vi "Station1_Data_Log.vi"(8 "error in (no error)":errorcluster, 10 "Parameters cluster":T3, 11 "Cluster":T2) -> (0 "error out":errorcluster)   [LabVIEW 2017]
uses:
  <vilib>/addons/database/Connection.llb/Conn ObjectReference.ctl
  <vilib>/addons/database/NI_Database_API.lvlib
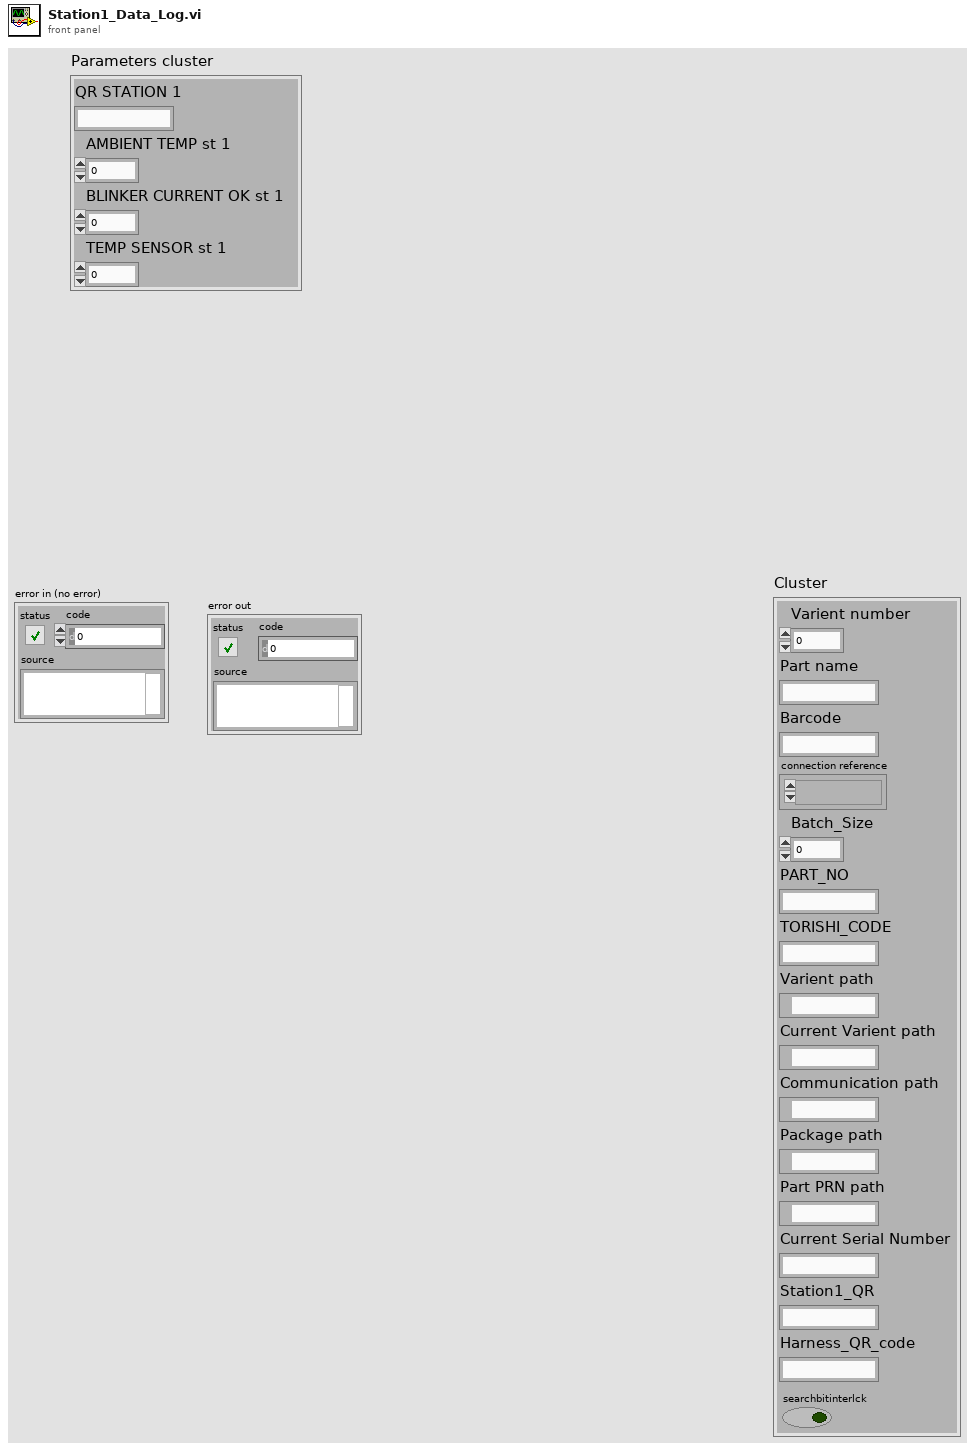
[diagram p1: front panel]
types:
  T1 = typedef "NI_Database_API.lvlib/Conn ObjectReference.ctl" = refnum<k1>
  T2 = cluster{"Varient number":u16, "Part name":string, "Barcode":string, "connection reference":T1, "Batch_Size":u16, "PART_NO":string, "TORISHI_CODE":string, "Varient path":path, "Current Varient path":path, "Communication path":path, "Package path":path, "Part PRN path":path, "Current Serial Number":string, "Station1_QR":string, "Harness_QR_code":string, "searchbitinterlck":bool}
  T3 = cluster{"QR STATION 1":string, "AMBIENT TEMP st 1":u32, "BLINKER CURRENT OK st 1":u32, "TEMP SENSOR st 1":u32}
  T4 = typedef "LVDateTimeRec.ctl" = cluster{"fractional second":dbl, "second":i32, "minute":i32, "hour":i32, "day of month":i32, "month":i32, "year":i32, "day of week":i32, "day of year":i32, "DST":i32}
  T5 = cluster{"time stamp":timestamp, string, string, "QR STATION 1":string, "Part name":string, "PART_NO":string, "TORISHI_CODE":string, string, string, "Current Serial Number":string, "Station1_QR":string, string, string, "Numeric 2":string, string, "Numeric 2":string, "Numeric 2":string, string, string, "Numeric 2":string, "Numeric 2":string, string, string, string, string, string, string, string, string, string, string, string, string}
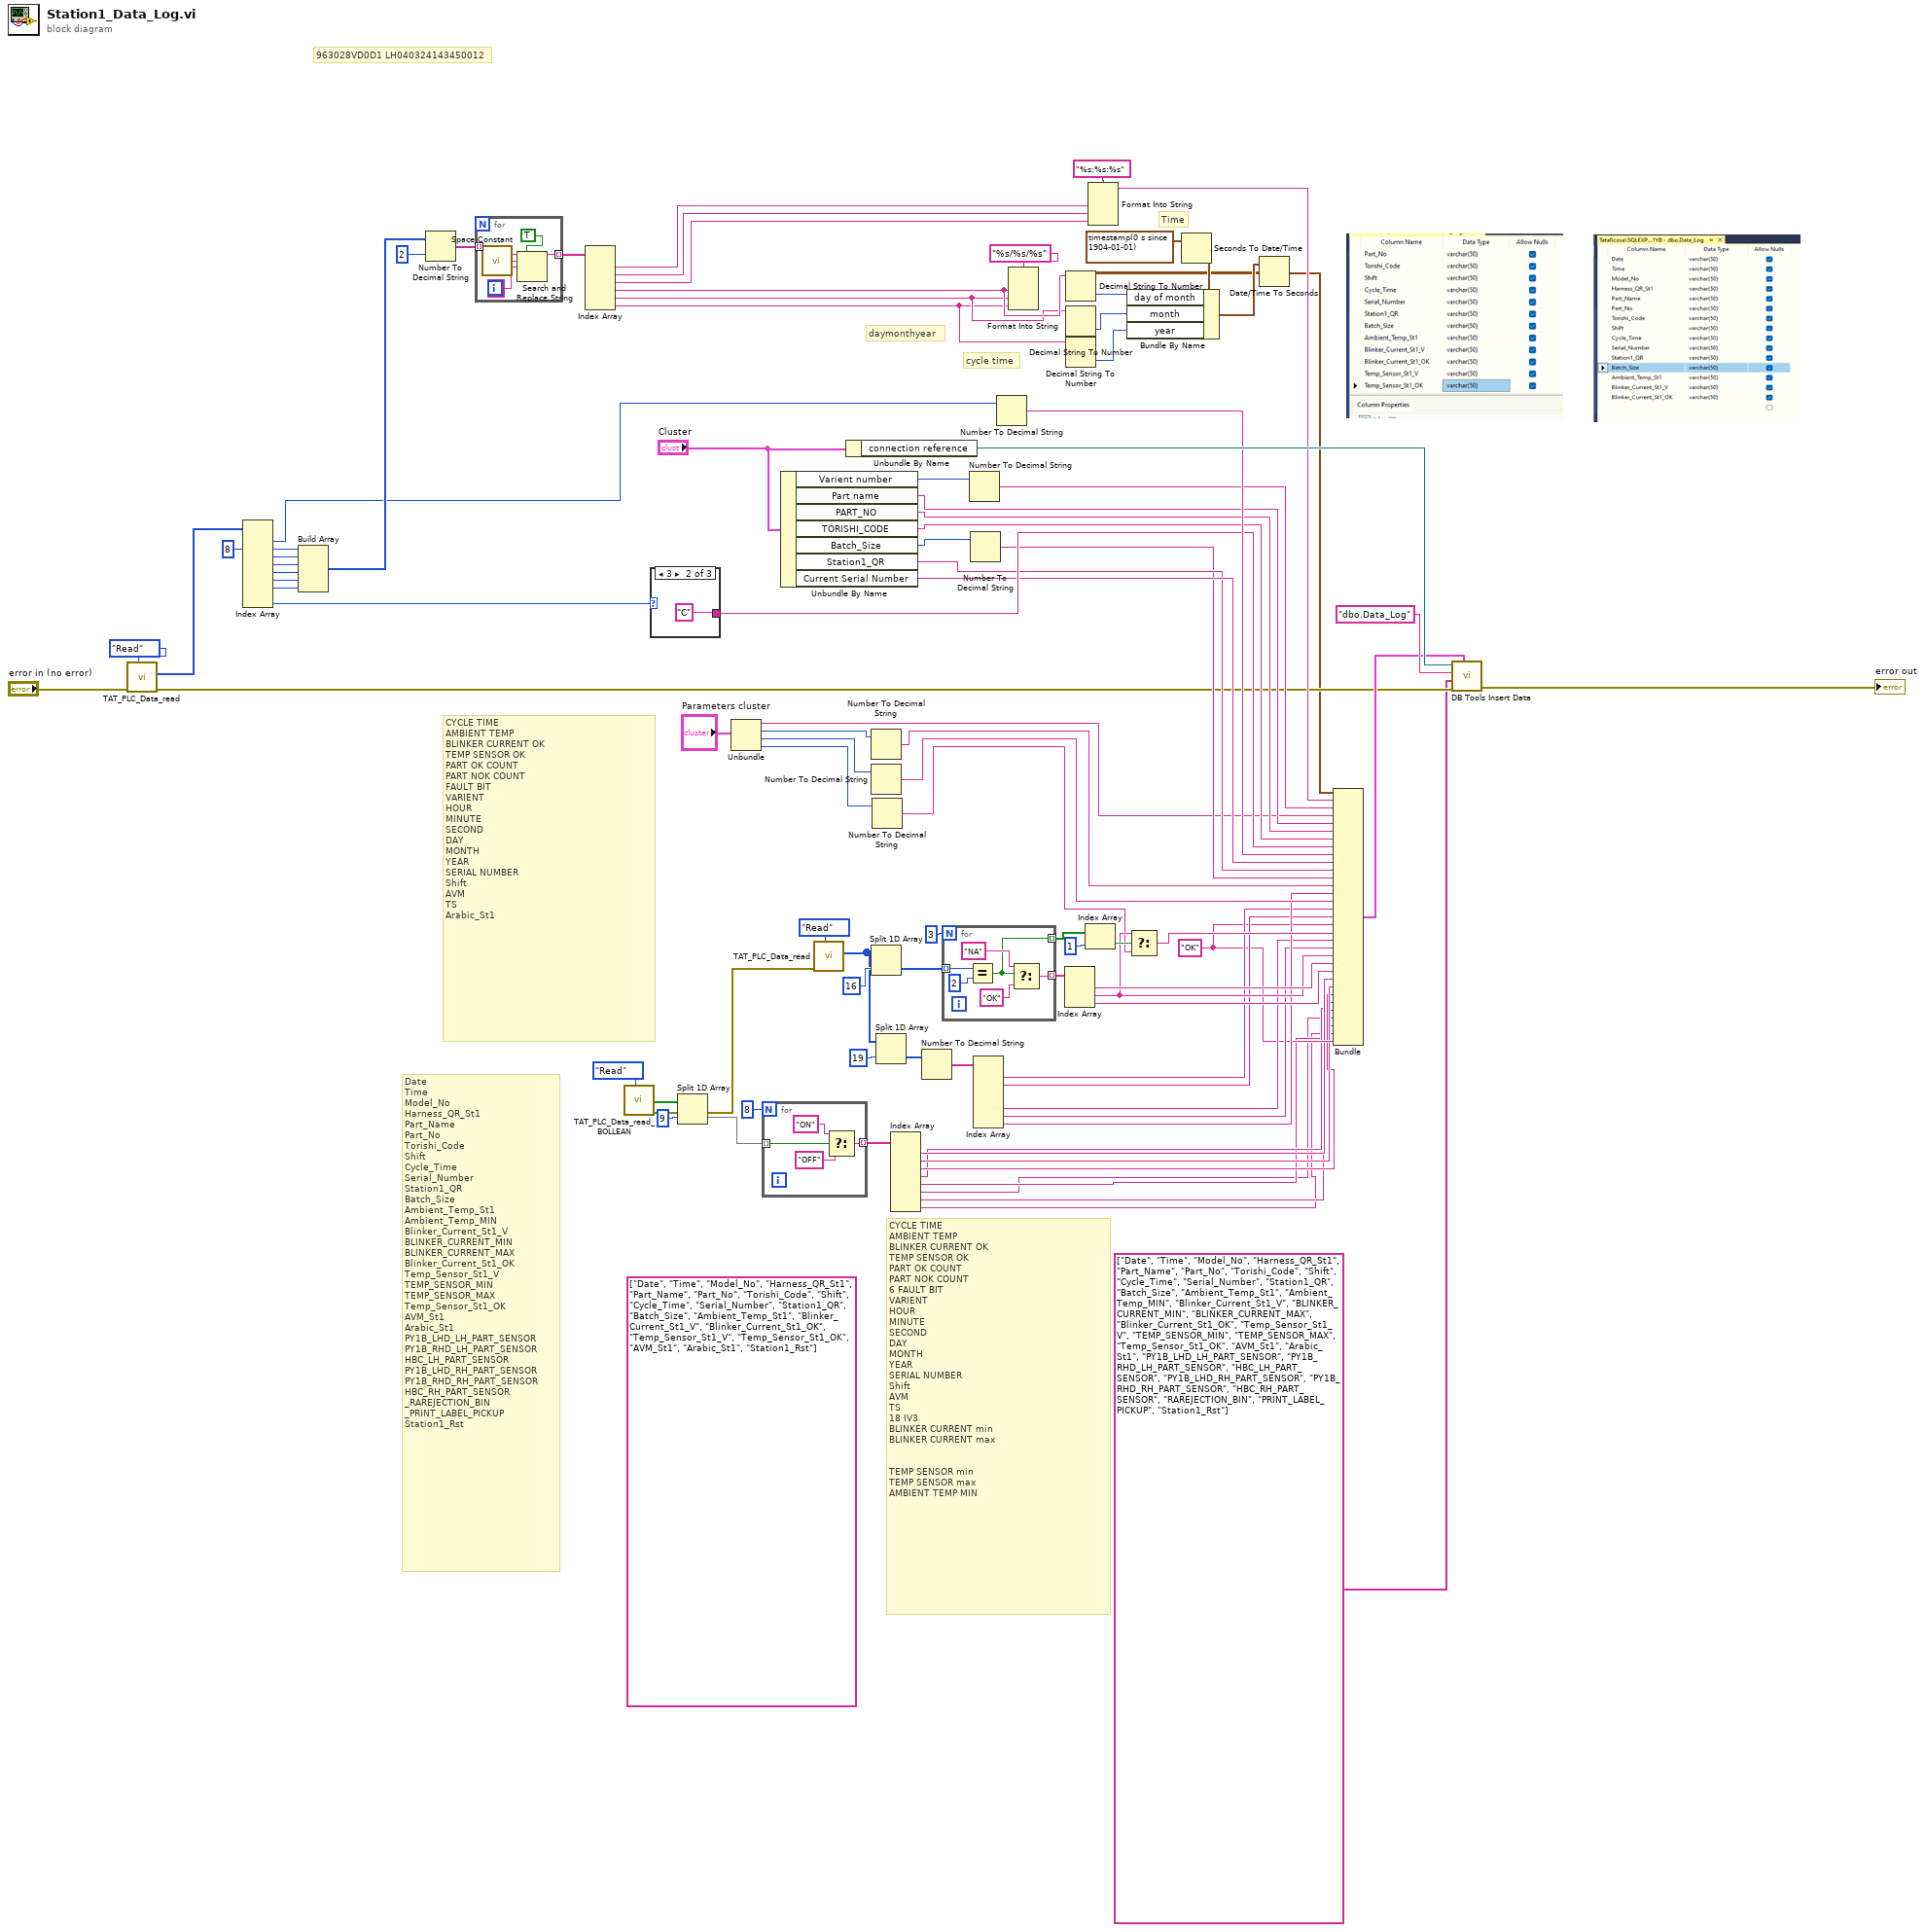
[diagram p0: block diagram]
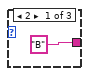
[diagram p2: hidden frame]
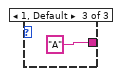
[diagram p3: hidden frame]
diagram:
  w26 = "OK"
  (unwired) string[] ["Date", "Time", "Model_No", "Harness_QR_St1", "Part_Name", "Part_No", "Torishi_Code", "Shift", "Cycle_Time", "Serial_Number", "Station1_QR", "Batch_Size", "Ambient_Temp_St1", "Blinker_Current_St1_V", "Blinker_Current_St1_OK", "Temp_Sensor_St1_V", "Temp_Sensor_St1_OK", "AVM_St1", "Arabic_St1", "Station1_Rst"] ("columns")
  # "Time"
  # "CYCLE TIME\nAMBIENT TEMP\nBLINKER CURRENT OK\nTEMP SENSOR OK\nPART OK COUNT\nPART NOK COUNT\n6 FAULT BIT\nVARIENT\nHOUR\nMINUTE\nSECOND\nDAY\nMONTH\nYEAR\nSERIAL NUMBER\nShift\nAVM\nTS\n18 IV3\nBLINKER CURRENT min\nBLINKER CURRENT max\n\n\nTEMP SENSOR min\nTEMP SENSOR max\nAMBIENT TEMP MIN"
  # "Date\nTime\nModel_No\nHarness_QR_St1\nPart_Name\nPart_No\nTorishi_Code\nShift\nCycle_Time\nSerial_Number\nStation1_QR\nBatch_Size\nAmbient_Temp_St1\nAmbient_Temp_MIN\nBlinker_Current_St1_V\nBLINKER_CURRENT_MIN\nBLINKER_CURRENT_MAX\nBlinker_Current_St1_OK\nTemp_Sensor_St1_V\nTEMP_SENSOR_MIN\nTEMP_SENSOR_MAX\nTemp_Sensor_St1_OK\nAVM_St1\nArabic_St1\nPY1B_LHD_LH_PART_SENSOR\nPY1B_RHD_LH_PART_SENSOR\nHBC_LH_PART_SENSOR\nPY1B_LHD_RH_PART_SENSOR\nPY1B_RHD_RH_PART_SENSOR\nHBC_RH_PART_SENSOR\n_RAREJECTION_BIN\n_PRINT_LABEL_PICKUP\nStation1_Rst"
  # "CYCLE TIME\nAMBIENT TEMP\nBLINKER CURRENT OK\nTEMP SENSOR OK\nPART OK COUNT\nPART NOK COUNT\nFAULT BIT\nVARIENT\nHOUR\nMINUTE\nSECOND\nDAY\nMONTH\nYEAR\nSERIAL NUMBER\nShift\nAVM\nTS\nArabic_St1"
  # "daymonthyear"
  # "963028VD0D1 LH040324143450012"
  # "cycle time"
  n1 = call "TAT_PLC_Data_read.vi"("Enum"=enum16{"Read", "Write"}."Read", "error in (no error)"="error in (no error)") -> ("error out"=w39:errorcluster, "Array 2"=w70:u16[])  [unwired: 8 in]
  n2 = Index Array(array=w70, index #2=8 ("index")) -> (element #1=w40:u16, element #2=w77:u16, element #3=w76:u16, element #4=w75:u16, element #5=w74:u16, element #6=w73:u16, element #7=w72:u16, element #9=w63:u16)  [unwired: 8 in, 1 out]
  n3 = Build Array(w77, w76, w75, w74, w73, w72) -> (w71:u16[])
  n4 = Number To Decimal String(number=w71, width (-)=i16 2) -> (decimal integer string=w80:string[])
  n5 = for {
    tunnel: w80 -> [w97] mode=indexing
    tunnel: [w96] -> w79 mode=indexing
    n6 = call <vilib>:"Space Constant.vi"() -> ("String"=w98:string)
    n7 = Search and Replace String(replace all?=TRUE ("replace all? (F)"), input string=w97, search string=w98, replace string="0" ("replace string (\"\")")) -> (result string=w96:string)  [unwired: 4 in, 3 out]
  }
  n8 = Index Array(array=w79) -> (element #1=w68:string, element #2=w67:string, element #3=w66:string, element #4=w3:string, element #5=w2:string, element #6=w1:string)  [unwired: 6 in]
  n9 = call "TAT_PLC_Data_read_BOLLEAN.vi"("Enum"=enum16{"Read", "Write"}."Read") -> ("error out"=w24:errorcluster, "Array 2"=w22:bool[])  [unwired: 9 in]
  n10 = case shown="3" w63 {
    tunnel: ["B" "C" "A"] -> w85
    frame 2 {
    }
    frame 3 {
    }
    frame 1, Default {
    }
  }
  n11 = Split 1D Array(array=w22, index=9) -> (second subarray=w20:bool[])  [unwired: 1 out]
  n12 = Unbundle("Parameters cluster") -> ("QR STATION 1"=w58:string, "AMBIENT TEMP st 1"=w57:u32, "BLINKER CURRENT OK st 1"=w56:u32, "TEMP SENSOR st 1"=w54:u32)
  n13 = for {
    N: 8 -> [_]
    tunnel: w20 -> [w105] mode=indexing
    tunnel: [w104] -> w19 mode=indexing
    n14 = Select(t="ON", s=w105, f="OFF") -> (s? t:f=w104:string)
  }
  n15 = Unbundle By Name("Cluster") -> ("Varient number"=w94:u16, "Part name"=w82:string, "PART_NO"=w88:string, "TORISHI_CODE"=w89:string, "Batch_Size"=w95:u16, "Station1_QR"=w61:string, "Current Serial Number"=w62:string)
  n16 = call "TAT_PLC_Data_read.vi"("Enum"=enum16{"Read", "Write"}."Read", "error in (no error)"=w24) -> ("Array 2"=w35:u16[])  [unwired: 8 in, 1 out]
  n17 = Unbundle By Name("Cluster") -> ("connection reference"=w93:T1)
  n18 = Number To Decimal String(number=w57) -> (decimal integer string=w36:string)  [unwired: 1 in]
  n19 = Number To Decimal String(number=w56) -> (decimal integer string=w55:string)  [unwired: 1 in]
  n20 = Split 1D Array(array=w35, index=16) -> (second subarray=w51:u16[])  [unwired: 1 out]
  n21 = Number To Decimal String(number=w54) -> (decimal integer string=w42:string)  [unwired: 1 in]
  n22 = Split 1D Array(array=w35, index=19) -> (second subarray=w33:u16[])  [unwired: 1 out]
  n23 = Index Array(array=w19) -> (element #1=w18:string, element #2=w17:string, element #3=w16:string, element #4=w15:string, element #5=w14:string, element #6=w13:string, element #7=w12:string, element #8=w11:string)  [unwired: 8 in]
  n24 = Number To Decimal String(number=w33) -> (decimal integer string=w32:string[])  [unwired: 1 in]
  n25 = for {
    N: 3 -> [_]
    tunnel: w51 -> [w113] mode=indexing
    tunnel: [w109] -> w49 mode=indexing
    tunnel: [w108] -> w45 mode=indexing
    n26 = Equal?(x=w113, y=2) -> (x = y?=w108:bool)
    n27 = Select(t="NA", s=w108, f="OK") -> (s? t:f=w109:string)
  }
  n28 = Number To Decimal String(number=w94) -> (decimal integer string=w87:string)  [unwired: 1 in]
  n29 = Number To Decimal String(number=w95) -> (decimal integer string=w60:string)  [unwired: 1 in]
  n30 = Index Array(array=w32) -> (element #1=w30:string, element #2=w29:string, element #5=w27:string, element #6=w28:string, element #7=w31:string)  [unwired: 7 in, 2 out]
  n31 = Number To Decimal String(number=w40) -> (decimal integer string=w90:string)  [unwired: 1 in]
  n32 = Format Into String(format string="%s/%s/%s" ("time format string (%c)"), w3, w2, w1) -> ()  [unwired: 2 in, 2 out]
  n33 = Index Array(array=w49) -> (element #1=w47:string, element #2=w43:string, element #3=w48:string)  [unwired: 3 in]
  n34 = Decimal String To Number(string=w3) -> (number=w7:i32)  [unwired: 2 in, 1 out]
  n35 = Decimal String To Number(string=w2) -> (number=w6:i32)  [unwired: 2 in, 1 out]
  n36 = Decimal String To Number(string=w1) -> (number=w5:i32)  [unwired: 2 in, 1 out]
  n37 = Index Array(array=w45, index=1) -> (element=w44:bool)
  n38 = Format Into String(format string="%s:%s:%s" ("time format string (%c)"), w68, w67, w66) -> (resulting string=w65:string)  [unwired: 2 in, 1 out]
  n39 = Select(t=w43, s=w44, f=w42) -> (s? t:f=w41:string)
  n40 = Seconds To Date/Time(time stamp (now)=timestamp(0 s since 1904-01-01)) -> (date time rec=w10:T4)  [unwired: 1 in]
  n41 = Bundle By Name(cluster=w10, "day of month"=w7, "month"=w6, "year"=w5) -> (w9:T4)
  n42 = Date/Time To Seconds(2:w9) -> (0:w4:timestamp)  [unwired: 1 in]
  n43 = Bundle("time stamp"=w4, w65, w87, "QR STATION 1"=w58, "Part name"=w82, "PART_NO"=w88, "TORISHI_CODE"=w89, w85, w90, "Current Serial Number"=w62, "Station1_QR"=w61, w60, w36, "Numeric 2"=w31, w55, "Numeric 2"=w30, "Numeric 2"=w29, w26, w41, "Numeric 2"=w27, "Numeric 2"=w28, w43, w47, w48, w18, w17, w16, w15, w14, w13, w12, w11, w26) -> (w86:T5)  [unwired: 1 in]
  n44 = call <vilib>:"DB Tools Insert Data.vi"("data"=w86, "error in (no error)"=w39, "columns"=string[] ["Date", "Time", "Model_No", "Harness_QR_St1", "Part_Name", "Part_No", "Torishi_Code", "Shift", "Cycle_Time", "Serial_Number", "Station1_QR", "Batch_Size", "Ambient_Temp_St1", "Ambient_Temp_MIN", "Blinker_Current_St1_V", "BLINKER_CURRENT_MIN", "BLINKER_CURRENT_MAX", "Blinker_Current_St1_OK", "Temp_Sensor_St1_V", "TEMP_SENSOR_MIN", "TEMP_SENSOR_MAX", "Temp_Sensor_St1_OK", "AVM_St1", "Arabic_St1", "PY1B_LHD_LH_PART_SENSOR", "PY1B_RHD_LH_PART_SENSOR", "HBC_LH_PART_SENSOR", "PY1B_LHD_RH_PART_SENSOR", "PY1B_RHD_RH_PART_SENSOR", "HBC_RH_PART_SENSOR", "RAREJECTION_BIN", "PRINT_LABEL_PICKUP", "Station1_Rst"], "table"="dbo.Data_Log", "connection reference"=w93) -> ("error out"=→"error out":errorcluster)  [unwired: 5 in, 1 out]
